vi "EEC EST 300 Run Test and Collect Data.vi"(8 "error in (no error)":errorcluster, 11 "VISA resource name":refnum<visa-resource-name>) -> (0 "error out":errorcluster, 2 "Read all Buffer":T2(array[cluster]), 3 "Test Data Cluster":T3)   [LabVIEW 2016]
doc: "This VI is an example to start a TEST, check the status of the test, and record data after a test. It is required that \"Saving and Creating a file\" is run before this."
uses:
  <instrlib>/eec EST 300/Public/Configure/Steps/Low Level/Test Type.ctl
  <instrlib>/eec EST 300/eec EST 300.lvlib
panel:
  in  "Step Number (1)":i32=1
  in  "Next Button":bool
  in  "Fail Stop On/OFF (F:Off)":bool
  in  "Single Step On/OFF (F:Off)":bool
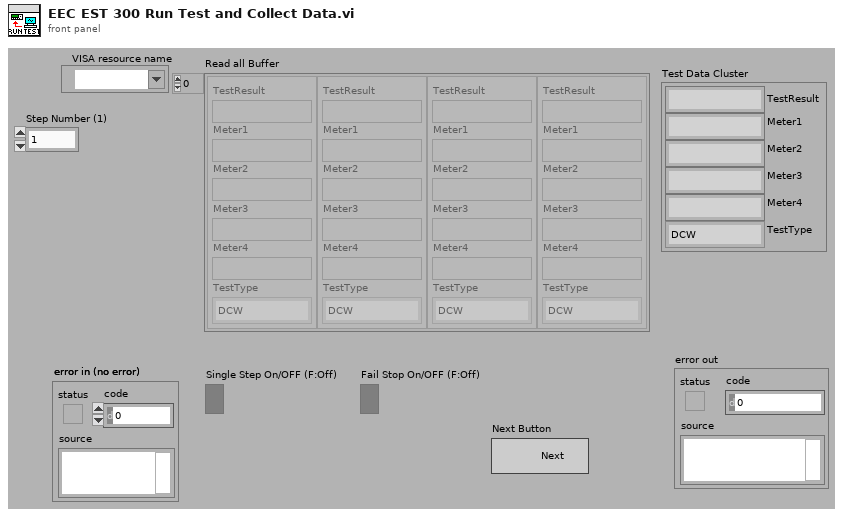
[diagram p1: front panel]
types:
  T1 = typedef "eec EST 300.lvlib/Test Type.ctl" = enum16{"DCW", "IR", "ACW"}
  T2 = cluster{"TestResult":string, "Meter1":string, "Meter2":string, "Meter3":string, "Meter4":string, "TestType":T1}[]
  T3 = cluster{"TestResult":string, "Meter1":string, "Meter2":string, "Meter3":string, "Meter4":string, "TestType":T1}
  T4 = cluster{"All Pass":bool, "Fail":bool, "Abort":bool, "Test in Process":bool, "Message Available":bool, "Event Summary Bit":bool, "Not Used":bool, "Prompt":bool}
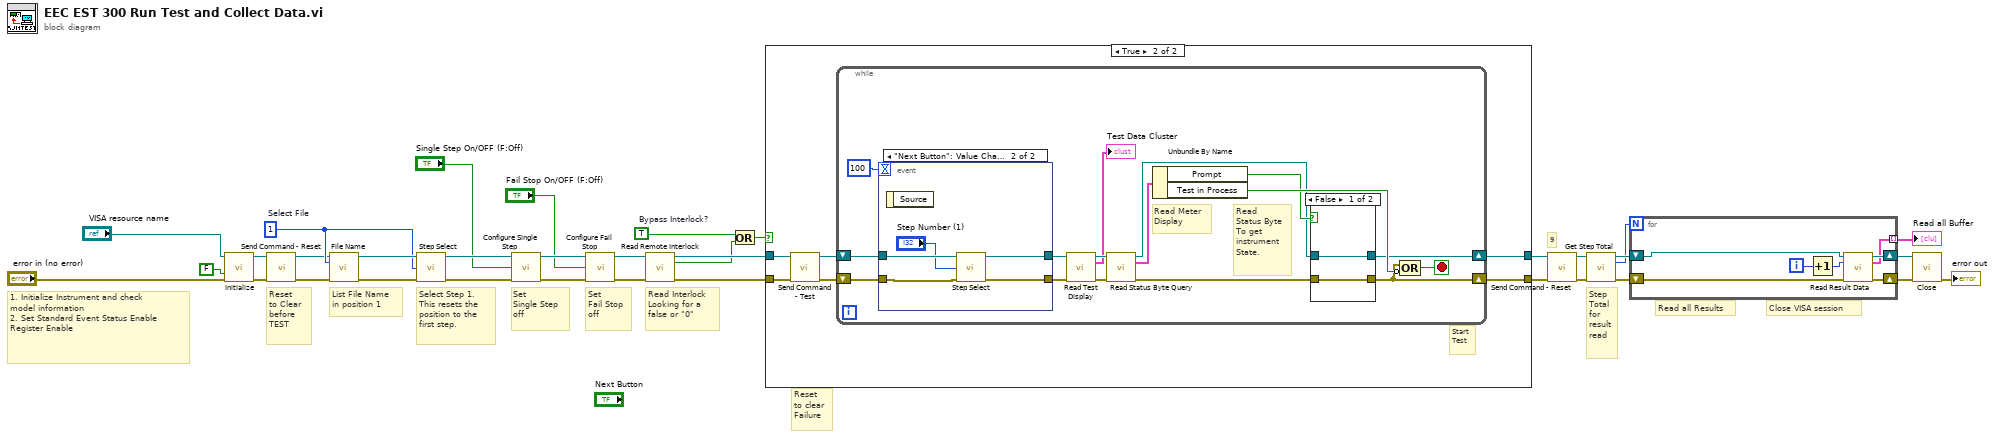
[diagram p0: block diagram]
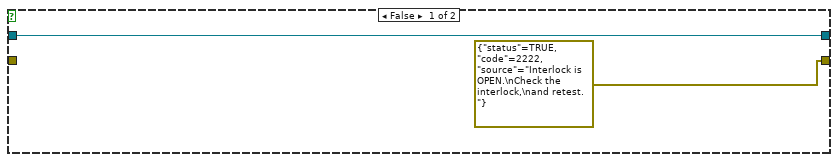
[diagram p2: hidden frame]
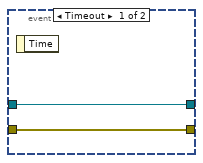
[diagram p3: hidden frame]
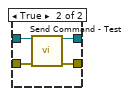
[diagram p4: hidden frame]
diagram:
  w6 = TRUE  # Bypass Interlock?
  w21 = 1  # Select File
  # "Close VISA session"
  # "Read all Results"
  # "Step\nTotal\nfor \nresult\nread"
  # "Reset\nto clear\nFailure"
  # "Read Interlock\nLooking for a\nfalse or \"0\""
  # "Set\nFail Stop\noff"
  # "Set \nSingle Step\noff"
  # "Select Step 1.\nThis resets the\nposition to the \nfirst step."
  # "List File Name\nin position 1"
  # "Reset\nto Clear \nbefore \nTEST"
  # "1. Initialize Instrument and check model information\n2. Set Standard Event Status Enable Register Enable"
  # "9"
  n1 = call <instrlib>:"Initialize.vi"("VISA resource name"="VISA resource name", "Reset (True)"=FALSE, "error in (no error)"="error in (no error)") -> ("VISA resource name out"=w5:refnum<visa-resource-name>, "error out"=w4:errorcluster)  [unwired: 10 in, 1 out]
  n2 = call <instrlib>:"Send Command - Reset.vi"("VISA resource name"=w5, "error in (no error)"=w4) -> ("VISA resource name out"=w12:refnum<visa-resource-name>, "error out"=w11:errorcluster)  [unwired: 12 in]
  n3 = call <instrlib>:"File Name.vi"("VISA resource name"=w12, "File Number"=w21, "error in (no error)"=w11) -> ("VISA resource name out"=w23:refnum<visa-resource-name>, "error out"=w22:errorcluster)  [unwired: 10 in, 1 out]
  n4 = call <instrlib>:"Step Select.vi"("VISA resource name"=w23, "Step Number (1)"=w21, "error in (no error)"=w22) -> ("VISA resource name out"=w20:refnum<visa-resource-name>, "error out"=w19:errorcluster)  [unwired: 11 in]
  n5 = call <instrlib>:"Configure Single Step.vi"("VISA resource name"=w20, "Single Step On/OFF (F:Off)"="Single Step On/OFF (F:Off)", "error in (no error)"=w19) -> ("VISA resource name out"=w18:refnum<visa-resource-name>, "error out"=w17:errorcluster)  [unwired: 11 in]
  n6 = call <instrlib>:"Configure Fail Stop.vi"("VISA resource name"=w18, "Fail Stop On/OFF (F:Off)"="Fail Stop On/OFF (F:Off)", "error in (no error)"=w17) -> ("VISA resource name out"=w15:refnum<visa-resource-name>, "error out"=w16:errorcluster)  [unwired: 11 in]
  n7 = call <instrlib>:"Read Remote Interlock.vi"("VISA resource name"=w15, "error in (no error)"=w16) -> ("VISA resource name out"=w14:refnum<visa-resource-name>, "Remote Interlock"=w10:bool, "error out"=w13:errorcluster)  [unwired: 11 in]
  n8 = Or(x=w6, y=w10) -> (x .or. y?=w7:bool)
  n9 = case shown="True" w7 {
    tunnel: [w36 w41] -> w34
    tunnel: [errorcluster {"status"=TRUE, "code"=2222, "source"="Interlock is OPEN.\nCheck the interlock,\nand retest."} ("error out") w40] -> w33
    tunnel: w14 -> [w36 w39]
    tunnel: w13 -> [_ w38]
    frame False {
    }
    frame True {
      # "Start\nTest"
      n10 = call <instrlib>:"Send Command - Test.vi"("VISA resource name"=w39, "error in (no error)"=w38) -> ("VISA resource name out"=w42:refnum<visa-resource-name>, "error out"=w37:errorcluster)  [unwired: 12 in]
      n11 = while {
        shift-left: w37 -> [w44]
        shift-right: [w54] -> w40
        shift-left: w42 -> [w46]
        shift-right: [w55] -> w41
        stop <- w58 stop-if-true
        # "Read Meter\nDisplay"
        # "Read \nStatus Byte\nTo get \ninstrument\nState."
        n12 = event shown="[1] \"Next Button\": Value Change" {
          selector: _ -> [_ _]
          dyn-events: _ -> [_ _]
          timeout: 100 -> [_ _]
          tunnel: [w60 w62] -> w47
          tunnel: w46 -> [w60 w65]
          tunnel: [w59 w61] -> w45
          tunnel: w44 -> [w59 w63]
          event Timeout {
            n13 = event-data() -> ()  [unwired: 1 in, 1 out]
          }
          event "Next Button": Value Change {
            n14 = event-data() -> ()  [unwired: 1 in, 1 out]
            n15 = call <instrlib>:"Step Select.vi"("VISA resource name"=w65, "Step Number (1)"="Step Number (1)", "error in (no error)"=w63) -> ("VISA resource name out"=w62:refnum<visa-resource-name>, "error out"=w61:errorcluster)  [unwired: 11 in]
          }
        }
        n16 = call <instrlib>:"Read Test Display.vi"("VISA resource name"=w47, "error in (no error)"=w45) -> ("VISA resource name out"=w50:refnum<visa-resource-name>, "Test Data Cluster"=→"Test Data Cluster":T3, "error out"=w49:errorcluster)  [unwired: 11 in]
        n17 = call <instrlib>:"Read Status Byte Query.vi"("VISA resource name"=w50, "error in (no error)"=w49) -> ("VISA resource name out"=w52:refnum<visa-resource-name>, "Status Byte Register"=w57:T4, "error out"=w51:errorcluster)  [unwired: 11 in]
        n18 = Unbundle By Name(w57) -> ("Prompt"=w53:bool, "Test in Process"=w56:bool)
        n19 = case shown="False" w53 {
          tunnel: w52 -> [w67 w71]
          tunnel: [w67 w70] -> w55
          tunnel: w51 -> [w66 w69]
          tunnel: [w66 w68] -> w54
          frame False {
          }
          frame True {
            n20 = call <instrlib>:"Send Command - Test.vi"("VISA resource name"=w71, "error in (no error)"=w69) -> ("VISA resource name out"=w70:refnum<visa-resource-name>, "error out"=w68:errorcluster)  [unwired: 12 in]
          }
        }
        n21 = Compound Arithmetic op=OR(w54, invert w56) -> (w58:bool)
      }
    }
  }
  n22 = call <instrlib>:"Send Command - Reset.vi"("VISA resource name"=w34, "error in (no error)"=w33) -> ("VISA resource name out"=w28:refnum<visa-resource-name>, "error out"=w27:errorcluster)  [unwired: 12 in]
  n23 = call <instrlib>:"Get Step Total.vi"("VISA resource name"=w28, "error in (no error)"=w27) -> ("VISA resource name out"=w26:refnum<visa-resource-name>, "# of Steps"=w24:i32, "error out"=w25:errorcluster)  [unwired: 11 in]
  n24 = for {
    N: w24 -> [_]
    shift-right: [w76] -> w9
    shift-left: w26 -> [w77]
    shift-right: [w74] -> w8
    shift-left: w25 -> [w72]
    tunnel: [w75] -> w3 mode=indexing
    i -> [w78]
    n25 = Increment(x=w78) -> (x+1=w73:i32)
    n26 = call <instrlib>:"Read Result Data.vi"("VISA resource name"=w77, "Result Number (1-200) (1)"=w73, "error in (no error)"=w72) -> ("VISA resource name out"=w76:refnum<visa-resource-name>, "Test Data Cluster"=w75:T3, "error out"=w74:errorcluster)  [unwired: 10 in]
  }
  "Read all Buffer" <- w3
  n27 = call <instrlib>:"Close.vi"("VISA resource name"=w9, "error in (no error)"=w8) -> ("error out"=→"error out":errorcluster)  [unwired: 13 in]
